vi "ini_load_variables.vi"(8 "error in":errorcluster, 10 "VI to store":refnum<vi>[](array[refnum]), 11 "objects to store":refnum<vi>[](array[refnum])) -> (0 "error out":errorcluster)   [LabVIEW 2018]
doc: "Loads referenced objects and controls of referenced VIs to INI file. Use this to load last setup of the programm."
uses:
  <vilib>/Utility/config.llb/NI_LVConfig.lvlib
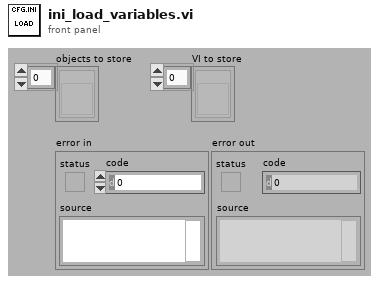
[diagram p1: front panel]
types:
  T1 = typedef "ini_parse_row.ctl" = cluster{"ini section":string, "ini key":string, "ini default":string, "control ref":refnum<vi>, "uid":i32, "vi ref":refnum<vi>}
  T2 = typedef "NI_LVConfig.lvlib/Config Data RefNum.ctl" = refnum<k1>
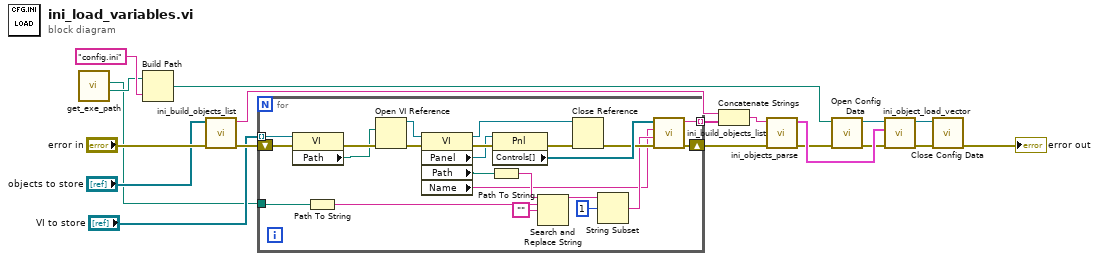
[diagram p0: block diagram]
diagram:
  n1 = call "get_exe_path.vi"() -> ("directory path"=w12:path, "application root path"=w1:path)  [unwired: 2 out]
  n2 = Build Path(base path=w12, name or relative path="config.ini") -> (appended path=w18:path)
  n3 = call "ini_build_objects_list.vi"("error in"="error in", "objects"="objects to store") -> ("error out"=w7:errorcluster, "objects list"=w3:string)  [unwired: 8 in]
  n4 = for {
    tunnel: "VI to store" -> [w36] mode=indexing
    shift-right: [w40] -> w5
    shift-left: w7 -> [w37]
    tunnel: [w38] -> w4 mode=indexing
    tunnel: w1 -> [w28]
    n5 = property class="VI"(reference=w36, error in=w37) -> (error out=w35:errorcluster, "Path"=w34:path)  [unwired: 1 out]
    n6 = Path To String(path=w28) -> (string=w25:string)
    n7 = Open VI Reference(vi path=w34, error in (no error)=w35) -> (vi reference=w32:refnum<vi>, error out=w33:errorcluster)  [unwired: 4 in]
    n8 = property class="VI"(reference=w32, error in=w33) -> (reference out=w29:refnum<vi>, error out=w42:errorcluster, "Panel"=w41:refnum<vi>, "Path"=w27:path, "Name"=w20:string)
    n9 = Path To String(path=w27) -> (string=w26:string)
    n10 = property class="Pnl"(reference=w41, error in=w42) -> (error out=w31:errorcluster, "Controls[]"=w39:refnum<vi>[])  [unwired: 1 out]
    n11 = Search and Replace String(input string=w26, search string=w25, replace string="" ("replace string (\"\")")) -> (result string=w23:string)  [unwired: 5 in, 3 out]
    n12 = Close Reference(reference=w29, error in (no error)=w31) -> (error out=w30:errorcluster)
    n13 = String Subset(string=w23, offset (0)=1) -> (substring=w21:string)  [unwired: 1 in]
    n14 = call "ini_build_objects_list.vi"("error in"=w30, "VI rel path (empty)"=w21, "VI name (empty)"=w20, "objects"=w39) -> ("error out"=w40:errorcluster, "objects list"=w38:string)  [unwired: 6 in]
  }
  n15 = Concatenate Strings(w3, w4) -> (w2:string)
  n16 = call "ini_objects_parse.vi"("error in"=w5, "items command"=w2) -> ("error out"=w9:errorcluster, "ini items"=w13:T1[])  [unwired: 8 in]
  n17 = call <vilib>:"Open Config Data.vi"("error in (no error)"=w9, "configuration file path"=w18) -> ("error out"=w8:errorcluster, "refnum"=w17:T2)  [unwired: 7 in, 1 out]
  n18 = call "ini_object_load_vector.vi"("error in"=w8, "objects to save"=w13, "refnum in"=w17) -> ("error out"=w16:errorcluster, "refnum out"=w15:T2)  [unwired: 7 in]
  n19 = call <vilib>:"Close Config Data.vi"("error in (no error)"=w16, "refnum"=w15) -> ("error out"=→"error out":errorcluster)  [unwired: 8 in, 1 out]
